vi "Alignment Main SLM.vi"   [LabVIEW 2014]
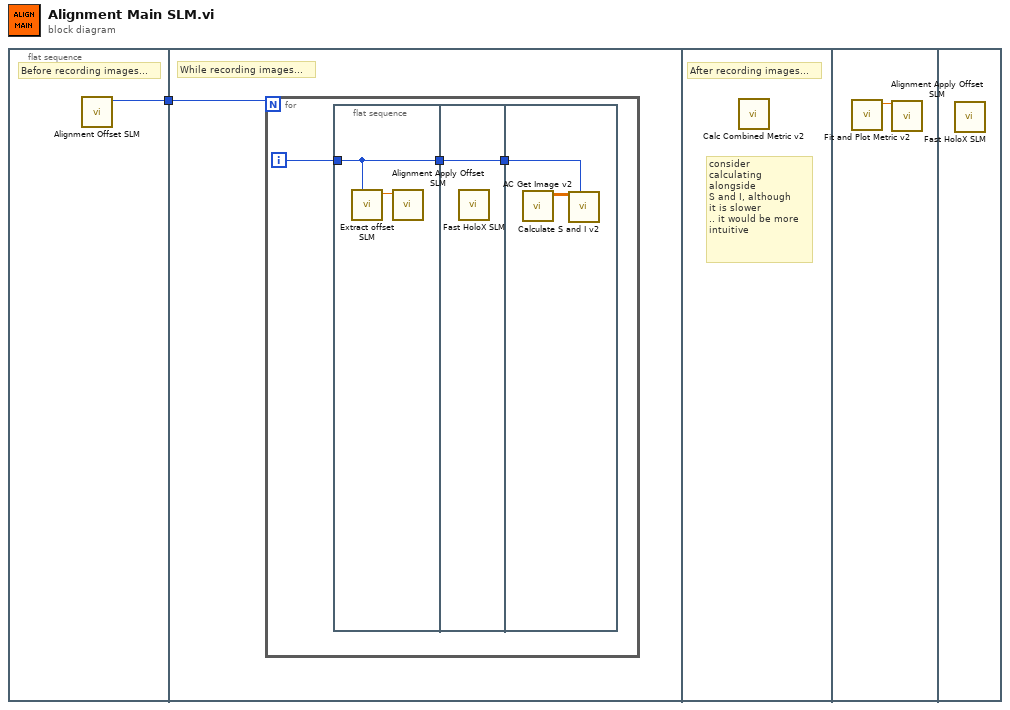
[diagram p0: block diagram]
diagram:
  n1 = flat-sequence {
    tunnel: [w2] -> w1
    tunnel: w1 -> [w3]
    frame #0 {
      # "Before recording images..."
      n2 = call "Alignment Offset SLM.vi"() -> ("number of steps align"=w2:u16)  [unwired: 11 in]
    }
    frame #1 {
      # "While recording images..."
      n3 = for {
        N: w3 -> [_]
        i -> [w6]
        n4 = flat-sequence {
          tunnel: w6 -> [w8]
          tunnel: [w8] -> w5
          tunnel: [w9] -> w4
          tunnel: w5 -> [w9]
          tunnel: w4 -> [w11]
          frame #0 {
            n5 = call "Extract offset SLM.vi"("current step index"=w8) -> ("current offset"=w7:dbl)  [unwired: 10 in]
            n6 = call "Alignment Apply Offset SLM.vi"("current offset"=w7) -> ()  [unwired: 11 in]
          }
          frame #1 {
            n7 = call "Fast HoloX SLM.vi"() -> ()  [unwired: 12 in]
          }
          frame #2 {
            n8 = call "AC Get Image v2.vi"() -> ("AC Image"=w10:sgl[][])  [unwired: 11 in]
            n9 = call "Calculate S and I v2.vi"("current step index"=w11, "AC Image"=w10) -> ()  [unwired: 10 in]
          }
        }
      }
    }
    frame #2 {
      # "consider\ncalculating\nalongside\nS and I, although\nit is slower\n.. it would be more \nintuitive"
      # "After recording images..."
      n10 = call "Calc Combined Metric v2.vi"() -> ()  [unwired: 12 in]
    }
    frame #3 {
      n11 = call "Fit and Plot Metric v2.vi"() -> ("Peak"=w12:dbl)  [unwired: 11 in]
      n12 = call "Alignment Apply Offset SLM.vi"("current offset"=w12) -> ()  [unwired: 11 in]
    }
    frame #4 {
      n13 = call "Fast HoloX SLM.vi"() -> ()  [unwired: 12 in]
    }
  }
